vi "Example Hello World.vi"() -> ()   [LabVIEW 2013]
uses:
  C:/tf/play/labview/Tinkerforge.dll
panel:
  in  "uid":string="SCD32"
  in  "port":i32=4223
  in  "host":string="localhost"
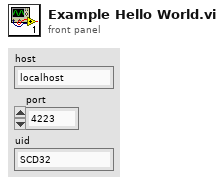
[diagram p1: front panel]
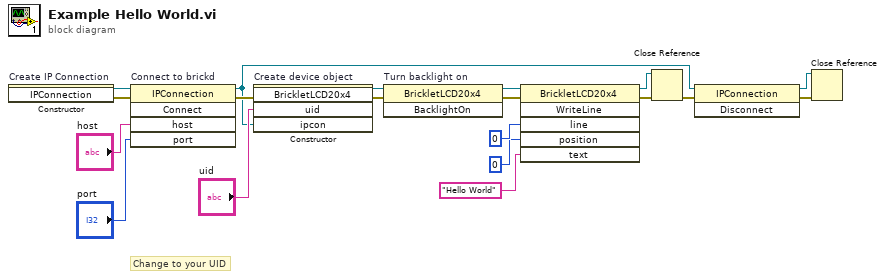
[diagram p0: block diagram]
diagram:
  # "Change to your UID"
  n1 = constructor on="Create IP Connection" class="IPConnection"() -> (reference out=w19:refnum<k24>, error out=w1:errorcluster)  [unwired: 3 in, 1 out]
  n2 = invoke on="Connect to brickd" class="IPConnection" method="Connect"(reference=w19, error in=w1, "host"="host", "port"="port") -> (reference out=w10:refnum<k24>, error out=w15:errorcluster)  [unwired: 1 in, 3 out]
  n3 = constructor on="Create device object" class="BrickletLCD20x4"(error in=w15, "uid"="uid", "ipcon"=w10) -> (reference out=w13:refnum<k24>, error out=w14:errorcluster)  [unwired: 2 in, 3 out]
  n4 = invoke on="Turn backlight on" class="BrickletLCD20x4" method="BacklightOn"(reference=w13, error in=w14) -> (reference out=w7:refnum<k24>, error out=w8:errorcluster)  [unwired: 1 in, 1 out]
  n5 = invoke class="BrickletLCD20x4" method="WriteLine"(reference=w7, error in=w8, "line"=u8 0, "position"=u8 0, "text"="Hello World") -> (reference out=w2:refnum<k24>, error out=w3:errorcluster)  [unwired: 1 in, 4 out]
  n6 = Close Reference(reference=w2, error in (no error)=w3) -> (error out=w12:errorcluster)
  n7 = invoke class="IPConnection" method="Disconnect"(reference=w10, error in=w12) -> (reference out=w9:refnum<k24>, error out=w11:errorcluster)  [unwired: 1 in, 1 out]
  n8 = Close Reference(reference=w9, error in (no error)=w11) -> ()  [unwired: 1 out]
